vi "test_Configure Response ByteCount.vi"(8 "error in (no error)":errorcluster, 11 "TestCase in":refnum<class "Instrument Addon Scripting API Messages Unit Tests.lvclass">) -> (0 "error out":errorcluster, 3 "TestCase out":refnum<class "Instrument Addon Scripting API Messages Unit Tests.lvclass">)   [LabVIEW 2019, in "Instrument Addon Scripting API Messages Unit Tests.lvclass"]
uses:
  Instrument Addon Scripting API Messages Unit Tests.lvclass
  <vilib>/addons/_JKI Toolkits/VI Tester/TestCase.llb/TestCase.lvclass
  APIs/Scripting API/Instrument Addon Scripting API.lvlib
  <vilib>/NI VeriStand/Custom Device API/Custom Device Item Ref.ctl
  <vilib>/NI VeriStand/Custom Device API/Custom Device API.lvlib
  APIs/Scripting API/TypeDefs/Linked Channel.ctl
  APIs/Scripting API/TypeDefs/ByteCount Response Settings.ctl
  Addon/Addon Shared/Types/FG Control.ctl
  Addon/Addon Shared/Instrument Addon Shared.lvlib
  <vilib>/NI/NI VeriStand Advanced SysDef API/SysDef API/Advanced System Definition.lvlib
  Addon/Addon Shared/SubVIs/Constants.vi
  <vilib>/NI/NI VeriStand Advanced SysDef API/_SubVIs/SysDef.Search.GUID.vi
  Addon/Addon Shared/Types/Linked Channel Cluster.ctl
  Addon/Addon Shared/Types/Response Wait Type.ctl
  Addon/Addon Shared/Types/Response Parameters.ctl
  APIs/Scripting API/Messages/Configure Response - Byte Count.vi
  C:/Program Files (x86)/National Instruments/LabVIEW 2019/vi.lib/addons/_JKI Toolkits/VI Tester/TestCase.llb/TestCase.lvclass
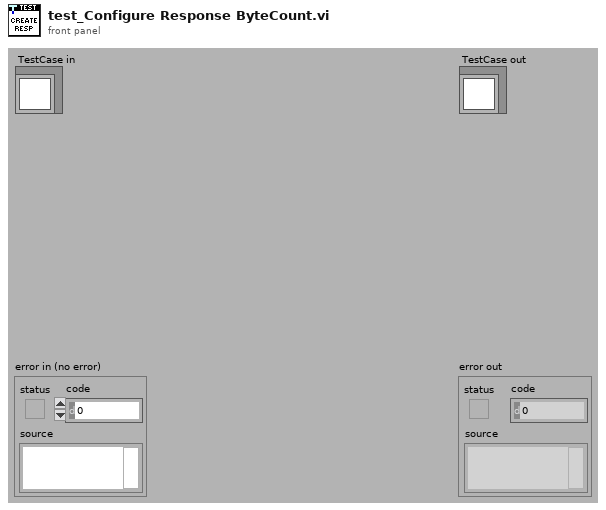
[diagram p1: front panel]
types:
  T1 = typedef "Instrument Addon Shared.lvlib/FG Control.ctl" = enum16{"Get", "Set"}
  T2 = typedef "Instrument Addon Scripting API.lvlib/ByteCount Response Settings.ctl" = cluster{"Response Format":string, "Linked Channels":T3[], "Byte Count":i32, "Use Byte Count channel":bool, "Channel Refnum":T4}
  T3 = typedef "Instrument Addon Scripting API.lvlib/Linked Channel.ctl" = cluster{"Variable Name":string, "Channel Refnum":T4}
  T4 = typedef "Custom Device API.lvlib/Custom Device Item Ref.ctl" = u64
  T5 = typedef "Instrument Addon Shared.lvlib/Response Parameters.ctl" = cluster{"Response":string, "Linked Channels":T6[], "Type Value":dbl, "Wait Type":T7, "Use Channel":bool, "Channel Path":string}
  T6 = typedef "Instrument Addon Shared.lvlib/Linked Channel Cluster.ctl" = cluster{"Variable Name":string, "GUID":string}
  T7 = typedef "Instrument Addon Shared.lvlib/Response Wait Type.ctl" = enum16{"Byte Count", "Wait sec"}
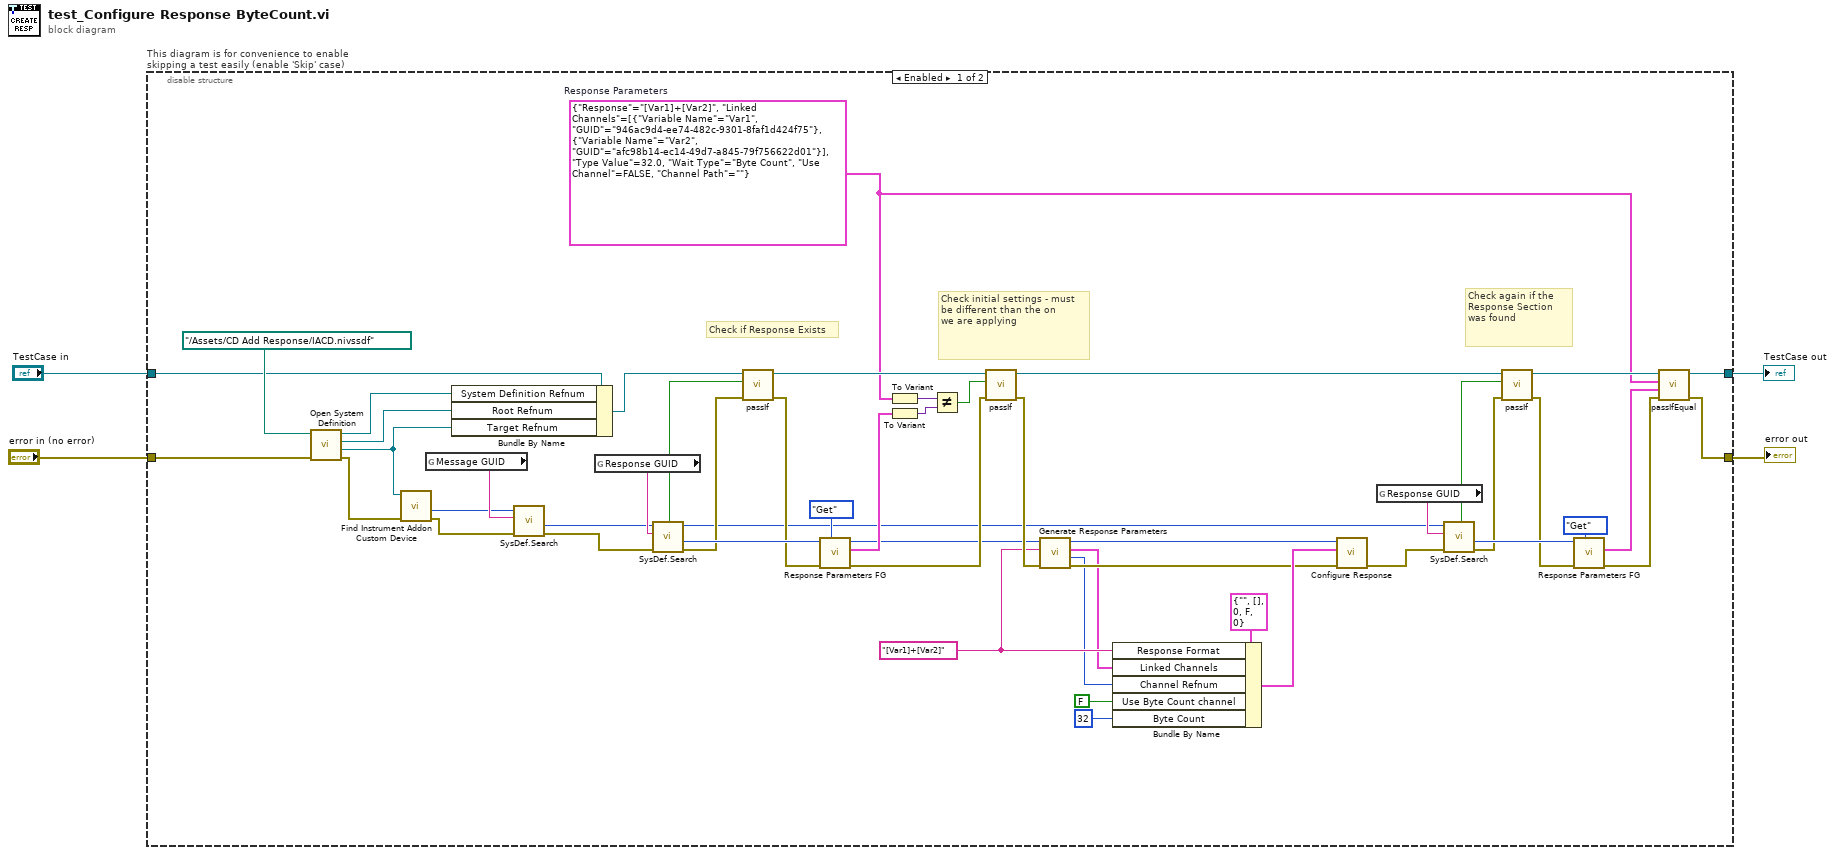
[diagram p0: block diagram]
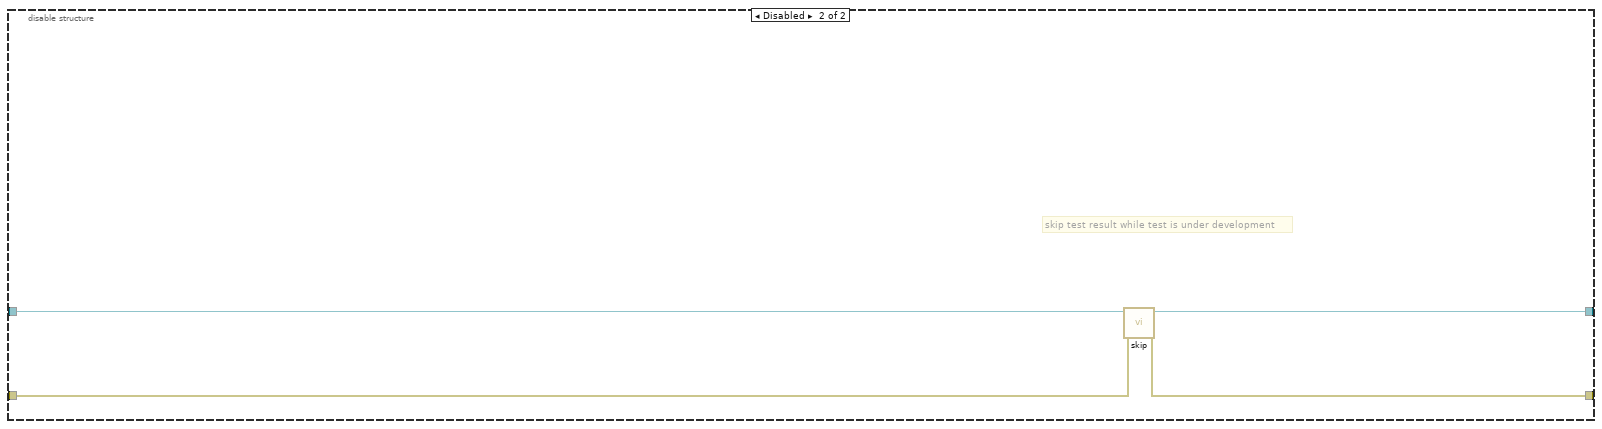
[diagram p2: hidden frame]
diagram:
  n1 = disable-structure "This diagram is for convenience to enable skipping a test easily (enable 'Skip' case)" shown="Enabled" {
    disable-tunnel: "TestCase in" -> [w12 w59]
    disable-tunnel: [w46 w57] -> w1
    disable-tunnel: [w45 w58] -> w3
    disable-tunnel: "error in (no error)" -> [w54 w56]
    frame Enabled {
      w22 = T5 {"Response"="[Var1]+[Var2]", "Linked Channels"=[{"Variable Name"="Var1", "GUID"="946ac9d4-ee74-482c-9301-8faf1d424f75"}, {"Variable Name"="Var2", "GUID"="afc98b14-ec14-49d7-a845-79f756622d01"}], "Type Value"=32.0, "Wait Type"=enum."Byte Count", "Use Channel"=FALSE, "Channel Path"=""}  # Response Parameters
      w17 = "[Var1]+[Var2]" ("Response Format")
      # "Check again if the Response Section was found"
      # "Check initial settings - must be different than the on\nwe are applying"
      # "Check if Response Exists"
      n2 = call "Open System Definition.vi"("error in (no error)"=w54, "System Definition File"=path "../Assets/CD Add Response/IACD.nivssdf" ("SDF file")) -> ("error out"=w53:errorcluster, "Target Refnum"=w10:refnum<k24>, "Root Refnum"=w9:refnum<k24>, "System Definition Refnum"=w8:refnum<k24>)  [unwired: 6 in]
      n3 = call "Find Instrument Addon Custom Device.vi"("error in"=w53, "target in"=w10) -> ("error out"=w27:errorcluster, "NodeID"=w24:u64)  [unwired: 7 in, 1 out]
      n4 = global read "Constants.vi" "Message GUID"() -> (w25:string)
      n5 = Bundle By Name(cluster=w12, "System Definition Refnum"=w8, "Root Refnum"=w9, "Target Refnum"=w10) -> (w11:refnum<class "Instrument Addon Scripting API Messages Unit Tests.lvclass">)
      n6 = call-poly <vilib>:"SysDef.Search.vi"("error in (no error)"=w27, "GUID"=w25, "nodeID"=w24) -> ("error out"=w26:errorcluster, "Value out"=w23:u64)  [unwired: 5 in, 2 out]
      n7 = global read "Constants.vi" "Response GUID"() -> (w42:string)
      n8 = call-poly <vilib>:"SysDef.Search.vi"("error in (no error)"=w26, "GUID"=w42, "nodeID"=w23) -> ("error out"=w35:errorcluster, "Value out"=w43:u64, "nodeID out"=w5:u64, "Found?"=w36:bool)  [unwired: 5 in]
      n9 = call-dynamic "passIf.vi"("error in (no error)"=w35, "pass"=w36, "TestCase in"=w11) -> ("error out"=w34:errorcluster, "TestCase out"=w33:refnum<class "Instrument Addon Scripting API Messages Unit Tests.lvclass">)  [unwired: 7 in]
      n10 = call "Response Parameters FG.vi"("Action"=FG_Control."Get", "error in (no error)"=w34, "Item Ref in"=w43) -> ("error out"=w21:errorcluster, "Response Parameters"=w41:T5, "Item Ref out"=w19:T4)  [unwired: 6 in]
      n11 = To Variant(anything=w22) -> (Variant=w40:variant)
      n12 = To Variant(anything=w41) -> (Variant=w39:variant)
      n13 = Not Equal?(x=w40, y=w39) -> (x != y?=w38:bool)
      n14 = call-dynamic "passIf.vi"("error in (no error)"=w21, "pass"=w38, "TestCase in"=w33) -> ("error out"=w20:errorcluster, "TestCase out"=w32:refnum<class "Instrument Addon Scripting API Messages Unit Tests.lvclass">)  [unwired: 7 in]
      n15 = call "Generate Response Parameters.vi"("Error In"=w20, "Response String"=w17, "Response Channel in"=w19) -> ("Error Out"=w18:errorcluster, "Wait Channel Ref out"=w15:T4, "Linked Channels"=w16:T3[], "Response Channel out"=w6:T4)  [unwired: 5 in]
      n16 = Bundle By Name(cluster=T2 {"Response Format"="", "Linked Channels"=[], "Byte Count"=0, "Use Byte Count channel"=FALSE, "Channel Refnum"=0} ("Settings"), "Response Format"=w17, "Linked Channels"=w16, "Channel Refnum"=w15, "Use Byte Count channel"=FALSE, "Byte Count"=32) -> (w51:T2)
      n17 = call-poly "Configure Response.vi"("error in (no error)"=w18, "settings"=w51, "response refnum in"=w6) -> ("error out"=w48:errorcluster)  [unwired: 7 in, 1 out]
      n18 = global read "Constants.vi" "Response GUID"() -> (w49:string)
      n19 = call-poly <vilib>:"SysDef.Search.vi"("error in (no error)"=w48, "GUID"=w49, "nodeID"=w5) -> ("error out"=w31:errorcluster, "Value out"=w47:u64, "Found?"=w30:bool)  [unwired: 5 in, 1 out]
      n20 = call-dynamic "passIf.vi"("error in (no error)"=w31, "pass"=w30, "TestCase in"=w32) -> ("error out"=w29:errorcluster, "TestCase out"=w28:refnum<class "Instrument Addon Scripting API Messages Unit Tests.lvclass">)  [unwired: 7 in]
      n21 = call "Response Parameters FG.vi"("Action"=FG_Control."Get", "error in (no error)"=w29, "Item Ref in"=w47) -> ("error out"=w7:errorcluster, "Response Parameters"=w37:T5)  [unwired: 6 in, 1 out]
      n22 = call-dynamic "passIfEqual.vi"("error in (no error)"=w7, "y"=w37, "x"=w22, "TestCase in"=w28) -> ("error out"=w45:errorcluster, "TestCase out"=w46:refnum<class "Instrument Addon Scripting API Messages Unit Tests.lvclass">)  [unwired: 6 in]
    }
    frame Disabled {
      # "skip test result while test is under development"
      n23 = call <vilib>:"skip.vi"("error in (no error)"=w56, "TestCase in"=w59) -> ("error out"=w58:errorcluster, "TestCase out"=w57:refnum<class "Instrument Addon Scripting API Messages Unit Tests.lvclass">)  [unwired: 8 in]
    }
  }
  "error out" <- w3
  "TestCase out" <- w1
